vi "Initialize DI.vi"(8 "error in (no error)":errorcluster, 9 "DI Channel Setting":T1, 10 "DAQ Type":enum16{"Hardware", "Simulation"}(ring), 11 "PXI 6515 in":refnum<class "PXI 6515.lvclass">) -> (0 "error out":errorcluster, 3 "PXI 6515 out":refnum<class "PXI 6515.lvclass">)   [LabVIEW 2021, in "DAQ IO.lvlib" / "PXI 6515.lvclass"]
uses:
  PXI 6515.lvclass
  DI Channel Setting.ctl
  PXI 6515.lvclass/PXI 6515.ctl
  DAQ IO.lvlib
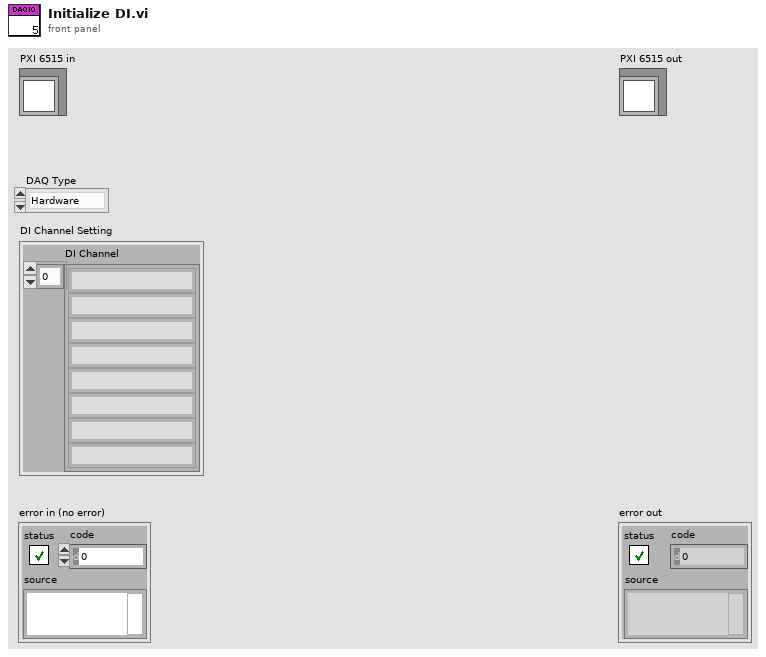
[diagram p1: front panel]
types:
  T1 = typedef "DAQ IO.lvlib/DI Channel Setting.ctl" = cluster{"DI Channel":string[]}
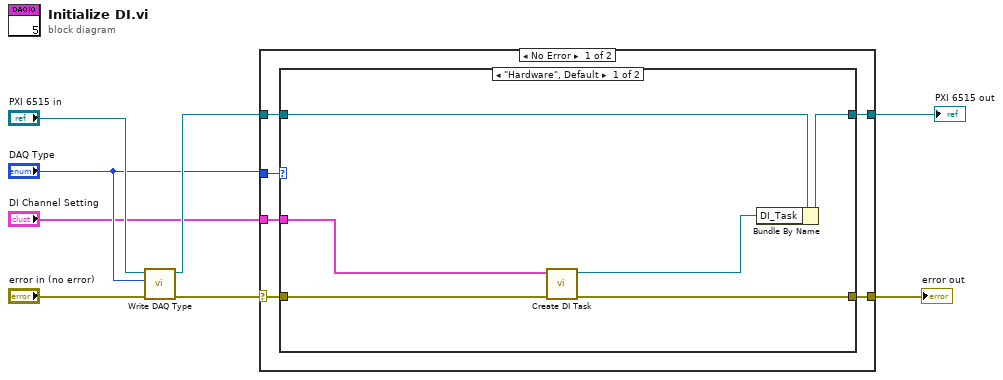
[diagram p0: block diagram]
diagram:
  n1 = call-dynamic "Write DAQ Type.vi"("error in (no error)"="error in (no error)", "DAQ Type"="DAQ Type", "PXI 6515 in"="PXI 6515 in") -> ("error out"=w7:errorcluster, "PXI 6515 out"=w5:refnum<class "PXI 6515.lvclass">)  [unwired: 7 in]
  n2 = case shown="No Error" w7 {
    selector: w7 -> [w13 w23]
    tunnel: w5 -> [w12 w24]
    tunnel: "DAQ Type" -> [w14 _]
    tunnel: [w11 w24] -> w3
    tunnel: [w10 w23] -> w2
    tunnel: "DI Channel Setting" -> [w9 _]
    frame No Error {
      n3 = case shown="\"Hardware\", Default" w14 {
        tunnel: w13 -> [w20 w21]
        tunnel: w12 -> [w18 w22]
        tunnel: [w17 w22] -> w11
        tunnel: [w19 w21] -> w10
        tunnel: w9 -> [w15 _]
        frame "Hardware", Default {
          n4 = call "Create DI Task.vi"("error in (no error)"=w20, "DI Channel Setting"=w15) -> ("error out"=w19:errorcluster, "DI_Task"=w16:refnum<k21>)  [unwired: 8 in]
          n5 = Bundle By Name(cluster=w18, "DI_Task"=w16) -> (w17:refnum<class "PXI 6515.lvclass">)
        }
        frame "Simulation" {
        }
      }
    }
    frame Error {
    }
  }
  "error out" <- w2
  "PXI 6515 out" <- w3
